vi "Testing WebDav folder finding.vi"() -> ()   [LabVIEW 2020]
uses:
  <vilib>/WebDAVClient/Advanced/FileInfo.ctl
  <vilib>/WebDAVClient/Advanced/Get Buffer.vi
  <vilib>/WebDAVClient/Advanced/Put Buffer.vi
  <vilib>/WebDAVClient/NI_WebDAV.lvlib
panel:
  out "data":string
  out "file list":T1[](array[typedef])
  out "directory list":T1[](array[typedef])
  out "error out":errorcluster
  out "local file path out":path
  in  "local file path":path
  out "x = y?":bool
  out "path 2":path
  out "String 2":string
  out "path":path
  in  "File Path":path
  out "String":string
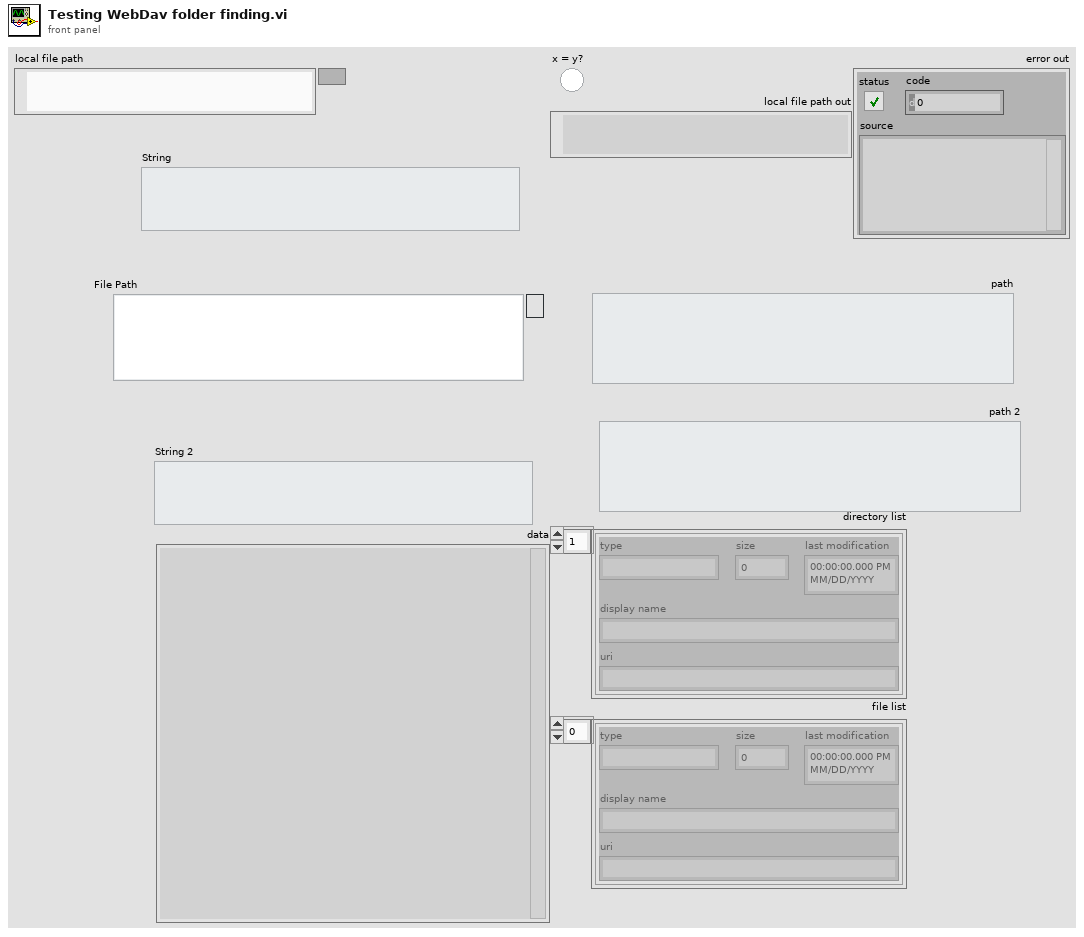
[diagram p1: front panel]
types:
  T1 = typedef "NI_WebDAV.lvlib/FileInfo.ctl" = cluster{"type":string, "size":u64, "last modification":timestamp, "display name":string, "uri":string}
  T2 = typedef "NI_WebDAV.lvlib/SessionHandle.ctl" = refnum<k1>
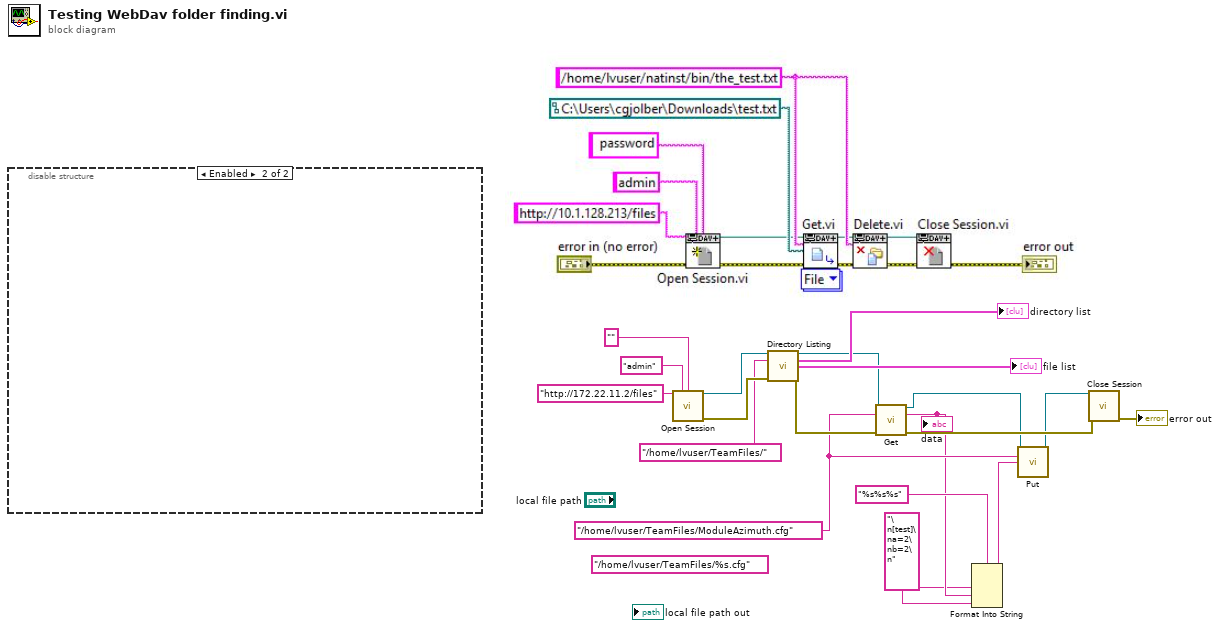
[diagram p0: block diagram]
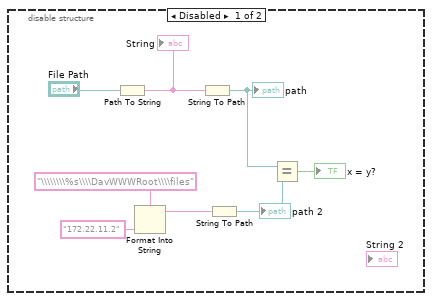
[diagram p2: hidden frame]
diagram:
  w1 = "\n[test]\na=2\nb=2\n" ("format string")
  w5 = "/home/lvuser/TeamFiles/ModuleAzimuth.cfg" ("relative uri")
  (unwired) "/home/lvuser/TeamFiles/%s.cfg" ("relative uri")
  n1 = disable-structure shown="Enabled" {
    frame Disabled {
      n2 = Path To String(path="File Path") -> (string=w26:string)
      "String" <- w26
      n3 = Format Into String(format string="\\\\\\\\%s\\\\DavWWWRoot\\\\files", "172.22.11.2" ("input 1")) -> (resulting string=w23:string)  [unwired: 2 in, 1 out]
      n4 = String To Path(string=w26) -> (path=w21:path)
      "path" <- w21
      n5 = String To Path(string=w23) -> (path=w22:path)
      "path 2" <- w22
      n6 = Equal?(x=w21, y=w22) -> (x = y?=→"x = y?":bool)
    }
    frame Enabled {
    }
  }
  n7 = call <vilib>:"Open Session.vi"("host uri prefix"="http://172.22.11.2/files", "username"="admin", "password"="") -> ("session handle out"=w15:T2, "error out"=w14:errorcluster)  [unwired: 11 in]
  n8 = call <vilib>:"Directory Listing.vi"("session handle"=w15, "relative uri"="/home/lvuser/TeamFiles/", "error in (no error)"=w14) -> ("session handle out"=w10:T2, "directory list"=→"directory list":T1[], "file list"=→"file list":T1[], "error out"=w9:errorcluster)  [unwired: 9 in]
  n9 = call-poly <vilib>:"Get.vi"("session handle"=w10, "relative uri"=w5, "error in (no error)"=w9) -> ("session handle out"=w7:T2, "data"=w2:string, "error out"=w8:errorcluster)  [unwired: 10 in]
  "data" <- w2
  n10 = Format Into String(format string="%s%s%s", w1, w2, w1) -> (resulting string=w3:string)  [unwired: 2 in, 1 out]
  n11 = call-poly <vilib>:"Put.vi"("session handle"=w7, "relative uri"=w5, "data"=w3) -> ("session handle out"=w6:T2)  [unwired: 11 in, 1 out]
  n12 = call <vilib>:"Close Session.vi"("session handle"=w6, "error in (no error)"=w8) -> ("error out"=→"error out":errorcluster)  [unwired: 13 in]
